vi "DeterminePuzzleMovements.vi"(10 "White Location In":T1, 11 "Peice Location In":T1) -> (0 "Upper White Row Position":i32, 1 "Current Peice Column":i32, 2 "Current Peice Row":i32, 3 "Lower White Column Position":i32, 5 "Allow Peice Movement":bool)   [LabVIEW 2014]
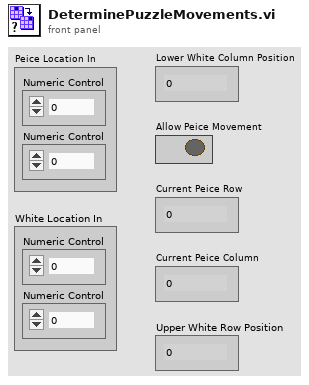
[diagram p1: front panel]
types:
  T1 = cluster{"Numeric Control":i32, "Numeric Control":i32}
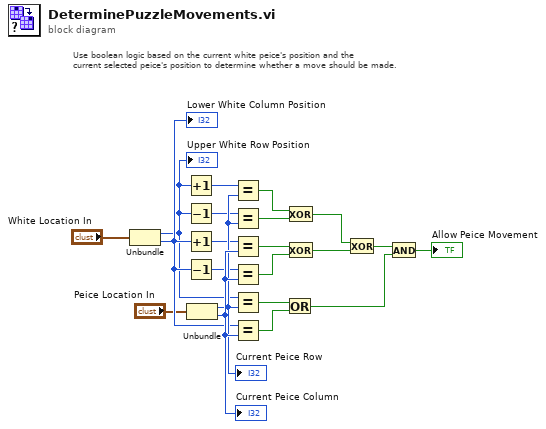
[diagram p0: block diagram]
diagram:
  # "Use boolean logic based on the current white peice's position and the\ncurrent selected peice's position to determine whether a move should be made."
  n1 = Unbundle("White Location In") -> ("Numeric Control"=w13:i32, "Numeric Control"=w14:i32)
  "Lower White Column Position" <- w14
  "Upper White Row Position" <- w13
  n2 = Increment(x=w13) -> (x+1=w3:i32)
  n3 = Decrement(x=w13) -> (x-1=w4:i32)
  n4 = Increment(x=w14) -> (x+1=w5:i32)
  n5 = Decrement(x=w14) -> (x-1=w6:i32)
  n6 = Unbundle("Peice Location In") -> ("Numeric Control"=w15:i32, "Numeric Control"=w16:i32)
  "Current Peice Column" <- w16
  "Current Peice Row" <- w15
  n7 = Equal?(x=w3, y=w15) -> (x = y?=w7:bool)
  n8 = Equal?(x=w4, y=w15) -> (x = y?=w8:bool)
  n9 = Equal?(x=w5, y=w16) -> (x = y?=w9:bool)
  n10 = Equal?(x=w6, y=w16) -> (x = y?=w10:bool)
  n11 = Equal?(x=w13, y=w15) -> (x = y?=w21:bool)
  n12 = Equal?(x=w14, y=w16) -> (x = y?=w20:bool)
  n13 = Or(x=w21, y=w20) -> (x .or. y?=w19:bool)
  n14 = Exclusive Or(1:w8, 2:w7) -> (0:w11:bool)
  n15 = Exclusive Or(1:w10, 2:w9) -> (0:w12:bool)
  n16 = Exclusive Or(1:w12, 2:w11) -> (0:w18:bool)
  n17 = And(x=w18, y=w19) -> (x .and. y?=→"Allow Peice Movement":bool)
